vi "BRig_RT__Case_Exp__State_RewardPre__v10.vi"(0 "input_dataCurrent":u16[](array[numeric]), 7 "input_dataExp":u16[](array[numeric]), 9 "input_dataBlock":u16[][](array[numeric]), 11 "input_dataTrial":u16[][](array[numeric])) -> (1 "output_T_Reward":u16, 2 "output_c_nReward_total_R":u16, 3 "output_c_nReward_total_L":u16, 4 "output_dataCurrent":u16[](array[numeric]), 6 "output_DAB_L=L":bool, 8 "output_DAB_R=HighPorb":bool, 10 "output_dataBlock":u16[][](array[numeric]), 13 "output_c_nReward_total":u16, 14 "output_nReward":u16, 15 "output_dataTrial":u16[][](array[numeric]))   [LabVIEW 2014]
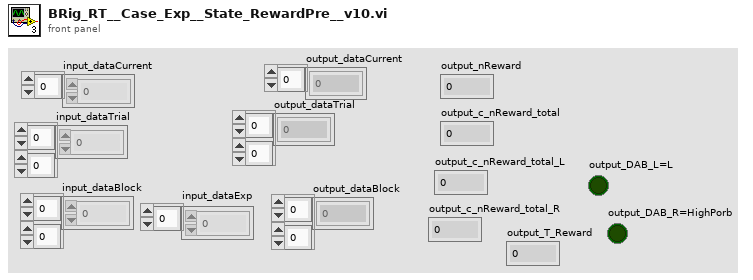
[diagram p1: front panel]
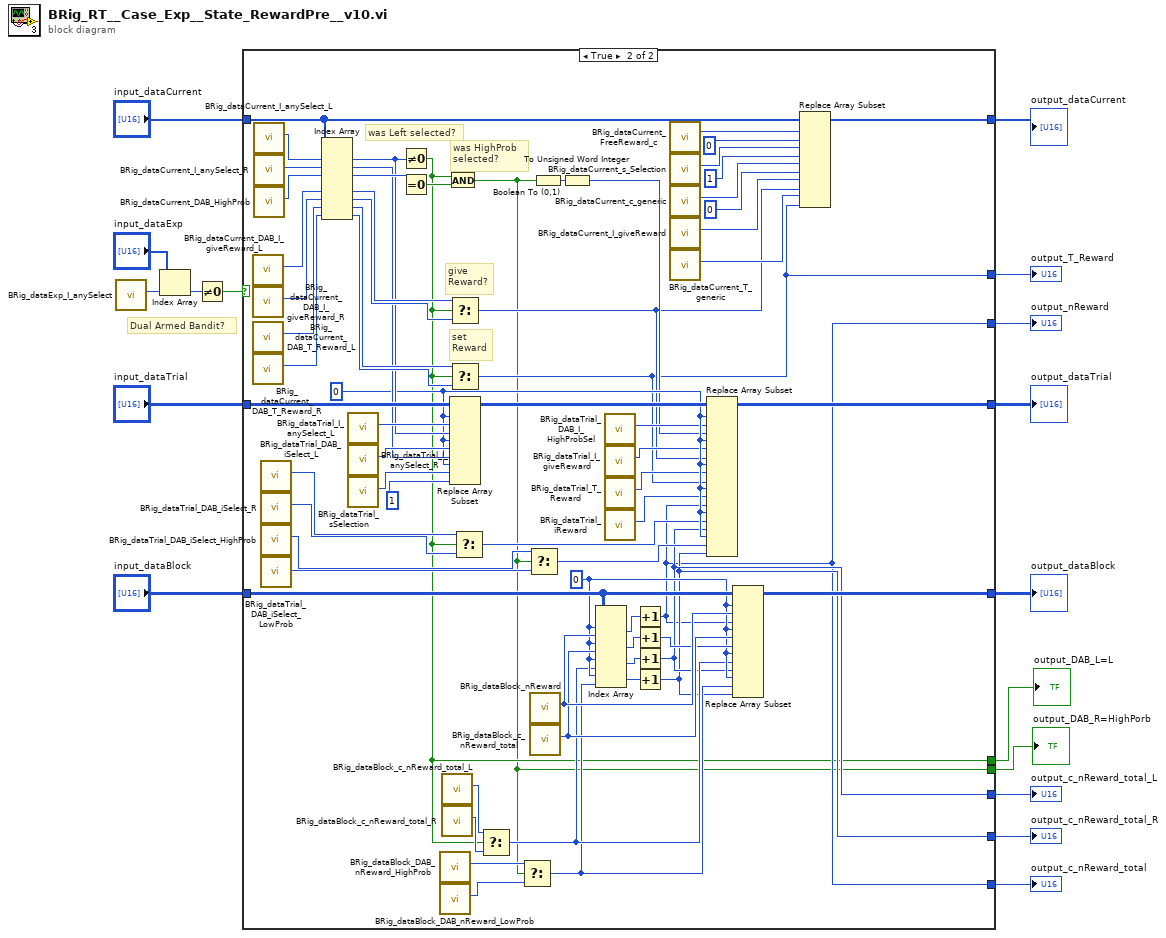
[diagram p0: block diagram]
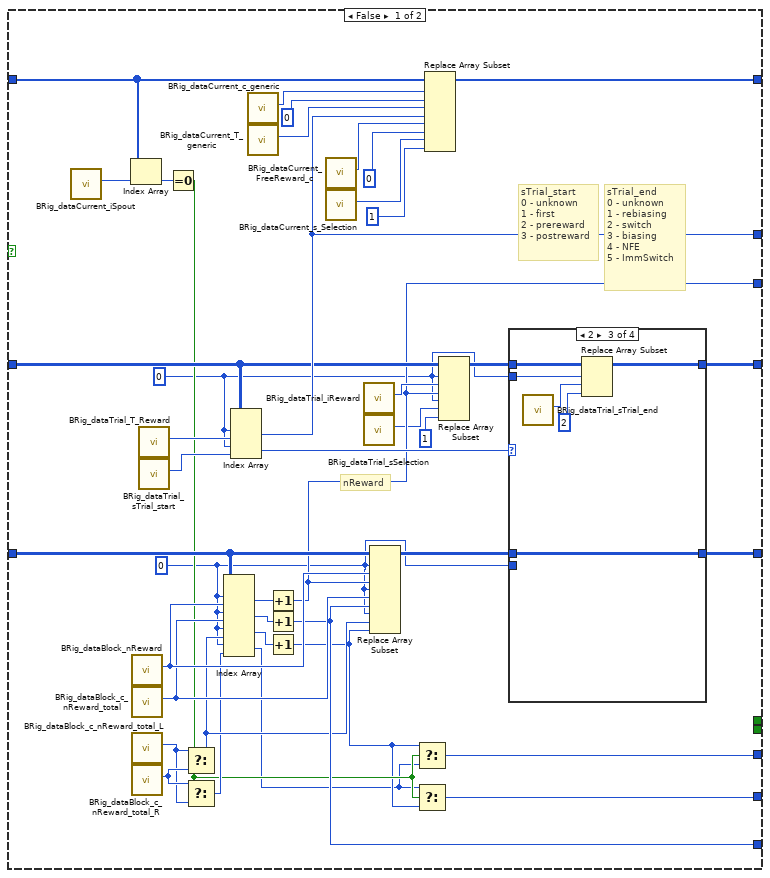
[diagram p2: hidden frame]
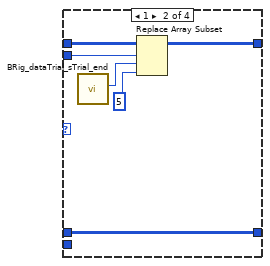
[diagram p4: hidden frame]
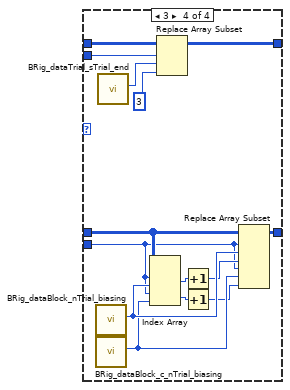
[diagram p5: hidden frame]
diagram:
  # "Dual Armed Bandit?"
  n1 = call "BRig_dataExp_I_anySelect.vi"() -> ("output_I_anySelect"=w10:i32)  [unwired: 11 in]
  n2 = Index Array(array="input_dataExp", index=w10) -> (element=w9:u16)
  n3 = Not Equal To 0?(x=w9) -> (x != 0?=w7:bool)
  n4 = case shown="True" w7 {
    tunnel: [w59 w155] -> w17
    tunnel: "input_dataCurrent" -> [w55 w146]
    tunnel: [w53 w93] -> w16
    tunnel: "input_dataBlock" -> [w52 w119]
    tunnel: [w47 w90] -> w15
    tunnel: "input_dataTrial" -> [w40 w128]
    tunnel: [w37 w90] -> w14
    tunnel: [w35 w116] -> w13
    tunnel: [w34 w117] -> w12
    tunnel: [w25 w92] -> w11
    tunnel: [w18 w91] -> w6
    tunnel: [_ w89] -> w2
    tunnel: [_ w88] -> w1
    frame False {
      w20 = 0
      w19 = 0
      # "nReward"
      # "sTrial_end\n0 - unknown\n1 - rebiasing\n2 - switch\n3 - biasing\n4 - NFE\n5 - ImmSwitch"
      # "sTrial_start\n0 - unknown\n1 - first\n2 - prereward\n3 - postreward"
      n5 = call "BRig_dataCurrent_iSpout.vi"() -> ("output_iSpout"=w46:i32)  [unwired: 11 in]
      n6 = Index Array(array=w55, index=w46) -> (element=w45:u16)
      n7 = call "BRig_dataBlock_nReward.vi"() -> ("output_nReward"=w51:i32)  [unwired: 11 in]
      n8 = call "BRig_dataBlock_c_nReward_total.vi"() -> ("output_nReward_total"=w48:i32)  [unwired: 11 in]
      n9 = call "BRig_dataBlock_c_nReward_total_L.vi"() -> ("output_nReward_total_L"=w30:i32)  [unwired: 11 in]
      n10 = call "BRig_dataBlock_c_nReward_total_R.vi"() -> ("output_nReward_total_R"=w31:i32)  [unwired: 11 in]
      n11 = call "BRig_dataTrial_T_Reward.vi"() -> ("output_T_Reward"=w54:i32)  [unwired: 11 in]
      n12 = call "BRig_dataTrial_sTrial_start.vi"() -> ("output_sTrial_start"=w42:i32)  [unwired: 11 in]
      n13 = Equal To 0?(x=w45) -> (x = 0?=w28:bool)
      n14 = Select(t=w30, s=w28, f=w31) -> (s? t:f=w43:i32)
      n15 = Select(t=w31, s=w28, f=w30) -> (s? t:f=w29:i32)
      n16 = Index Array(array=w52, index (row) #1=w19, index (col) #1=w51, index (row) #2=w19, index (col) #2=w48, index (row) #3=w19, index (col) #3=w43, index (row) #4=w19, index (col) #4=w29) -> (element #1=w50:u16, element #2=w49:u16, element #3=w44:u16, element #4=w26:u16)
      n17 = Index Array(array=w40, index (row) #1=w20, index (col) #1=w54, index (row) #2=w20, index (col) #2=w42) -> (element #1=w53:u16, element #2=w41:u16)
      n18 = call "BRig_dataCurrent_c_generic.vi"() -> ("output_count_generic"=w58:i32)  [unwired: 11 in]
      n19 = call "BRig_dataCurrent_T_generic.vi"() -> ("output_T_generic"=w57:i32)  [unwired: 11 in]
      n20 = Increment(x=w50) -> (x+1=w37:u16)
      n21 = Increment(x=w49) -> (x+1=w47:u16)
      n22 = Increment(x=w44) -> (x+1=w27:u16)
      n23 = call "BRig_dataCurrent_FreeReward_c.vi"() -> ("output_FreeReward_c"=w24:i32)  [unwired: 11 in]
      n24 = call "BRig_dataCurrent_s_Selection.vi"() -> ("output_s_Selection"=w22:i32)  [unwired: 11 in]
      n25 = call "BRig_dataTrial_iReward.vi"() -> ("output_iReward"=w38:i32)  [unwired: 11 in]
      n26 = call "BRig_dataTrial_sSelection.vi"() -> ("output_sSelection"=w33:i32)  [unwired: 11 in]
      n27 = Replace Array Subset(array=w52, new element #1=w37, index (row) #1=w19, index (col) #1=w51, new element #2=w47, index (row) #2=w19, index (col) #2=w48, new element #3=w27, index (row) #3=w19, index (col) #3=w43) -> (w36:u16[][])
      n28 = Select(t=w27, s=w28, f=w26) -> (s? t:f=w25:u16)
      n29 = Select(t=w26, s=w28, f=w27) -> (s? t:f=w18:u16)
      n30 = Replace Array Subset(array=w55, new element #1=u16 0 ("new element/subarray"), index #1=w58, new element #2=w53, index #2=w57, new element #3=u16 0 ("new element/subarray"), index #3=w24, new element #4=u16 1 ("new element/subarray"), index #4=w22) -> (w59:u16[])
      n31 = Replace Array Subset(array=w40, new element #1=w37, index (row) #1=w20, index (col) #1=w38, new element #2=u16 1 ("new element/subarray"), index (row) #2=w20, index (col) #2=w33) -> (w39:u16[][])
      n32 = case shown="2" w41 {
        tunnel: w39 -> [w61 w67 w73 w87]
        tunnel: w20 -> [_ w65 w71 w85]
        tunnel: [w61 w66 w72 w86] -> w34
        tunnel: w36 -> [w60 w62 w68 w81]
        tunnel: [w60 w62 w68 w82] -> w35
        tunnel: w19 -> [_ _ _ w77]
        frame 0, Default {
        }
        frame 1 {
          n33 = call "BRig_dataTrial_sTrial_end.vi"() -> ("output_sTrial_end"=w64:i32)  [unwired: 11 in]
          n34 = Replace Array Subset(array=w67, new element=u16 5 ("new element/subarray"), index (row)=w65, index (col)=w64) -> (w66:u16[][])
        }
        frame 2 {
          n35 = call "BRig_dataTrial_sTrial_end.vi"() -> ("output_sTrial_end"=w70:i32)  [unwired: 11 in]
          n36 = Replace Array Subset(array=w73, new element=u16 2 ("new element/subarray"), index (row)=w71, index (col)=w70) -> (w72:u16[][])
        }
        frame 3 {
          n37 = call "BRig_dataBlock_nTrial_biasing.vi"() -> ("output_nTrial_biasing"=w80:i32)  [unwired: 11 in]
          n38 = call "BRig_dataBlock_c_nTrial_biasing.vi"() -> ("output_c_nTrial_biasing"=w75:i32)  [unwired: 11 in]
          n39 = call "BRig_dataTrial_sTrial_end.vi"() -> ("output_sTrial_end"=w84:i32)  [unwired: 11 in]
          n40 = Index Array(array=w81, index (row) #1=w77, index (col) #1=w80, index (row) #2=w77, index (col) #2=w75) -> (element #1=w79:u16, element #2=w76:u16)
          n41 = Replace Array Subset(array=w87, new element=u16 3 ("new element/subarray"), index (row)=w85, index (col)=w84) -> (w86:u16[][])
          n42 = Increment(x=w79) -> (x+1=w78:u16)
          n43 = Increment(x=w76) -> (x+1=w74:u16)
          n44 = Replace Array Subset(array=w81, new element #1=w78, index (row) #1=w77, index (col) #1=w80, new element #2=w74, index (row) #2=w77, index (col) #2=w75) -> (w82:u16[][])
        }
      }
    }
    frame True {
      w115 = 0
      w102 = 0
      # "set\nReward"
      # "give\nReward?"
      # "was HighProb\nselected?"
      # "was Left selected?"
      n45 = call "BRig_dataCurrent_DAB_I_giveReward_L.vi"() -> ("output_DAB_I_giveReward_L"=w140:i32)  [unwired: 11 in]
      n46 = call "BRig_dataCurrent_DAB_I_giveReward_R.vi"() -> ("output_DAB_I_giveReward_R"=w139:i32)  [unwired: 11 in]
      n47 = call "BRig_dataCurrent_DAB_T_Reward_L.vi"() -> ("output_DAB_T_Reward_L"=w134:i32)  [unwired: 11 in]
      n48 = call "BRig_dataCurrent_DAB_T_Reward_R.vi"() -> ("output_DAB_T_Reward_R"=w133:i32)  [unwired: 11 in]
      n49 = call "BRig_dataCurrent_I_anySelect_L.vi"() -> ("output_IanySelect_L"=w145:i32)  [unwired: 11 in]
      n50 = call "BRig_dataCurrent_I_anySelect_R.vi"() -> ("output_IanySelect_R"=w144:i32)  [unwired: 11 in]
      n51 = call "BRig_dataCurrent_DAB_HighProb.vi"() -> ("output_DAB_HighProb"=w143:i32)  [unwired: 11 in]
      n52 = call "BRig_dataTrial_DAB_iSelect_L.vi"() -> ("output_DAB_iSelect_L"=w106:i32)  [unwired: 11 in]
      n53 = call "BRig_dataTrial_DAB_iSelect_R.vi"() -> ("output_DAB_iSelect_R"=w105:i32)  [unwired: 11 in]
      n54 = call "BRig_dataTrial_DAB_iSelect_HighProb.vi"() -> ("output_DAB_iSelect_HighProb"=w103:i32)  [unwired: 11 in]
      n55 = call "BRig_dataTrial_DAB_iSelect_LowProb.vi"() -> ("output_DAB_iSelect_LowProb"=w104:i32)  [unwired: 11 in]
      n56 = Index Array(array=w146, index #1=w145, index #2=w144, index #3=w143, index #5=w140, index #6=w139, index #7=w134, index #8=w133) -> (element #1=w127:u16, element #2=w126:u16, element #3=w142:u16, element #5=w138:u16, element #6=w137:u16, element #7=w136:u16, element #8=w135:u16)  [unwired: 1 in, 1 out]
      n57 = call "BRig_dataTrial_I_anySelect_L.vi"() -> ("output_I_allReward_L"=w132:i32)  [unwired: 11 in]
      n58 = call "BRig_dataTrial_I_anySelect_R.vi"() -> ("output_I_anySelect_R"=w131:i32)  [unwired: 11 in]
      n59 = call "BRig_dataTrial_sSelection.vi"() -> ("output_sSelection"=w130:i32)  [unwired: 11 in]
      n60 = Not Equal To 0?(x=w127) -> (x != 0?=w89:bool)
      n61 = Equal To 0?(x=w142) -> (x = 0?=w141:bool)
      n62 = call "BRig_dataBlock_DAB_nReward_HighProb.vi"() -> ("output_DAB_nReward_HighProb"=w112:i32)  [unwired: 11 in]
      n63 = call "BRig_dataBlock_DAB_nReward_LowProb.vi"() -> ("output_DAB_nReward_LowProb"=w111:i32)  [unwired: 11 in]
      n64 = call "BRig_dataBlock_c_nReward_total_L.vi"() -> ("output_nReward_total_L"=w114:i32)  [unwired: 11 in]
      n65 = call "BRig_dataBlock_c_nReward_total_R.vi"() -> ("output_nReward_total_R"=w113:i32)  [unwired: 11 in]
      n66 = And(x=w89, y=w141) -> (x .and. y?=w88:bool)
      n67 = Select(t=w138, s=w89, f=w137) -> (s? t:f=w94:u16)
      n68 = Select(t=w136, s=w89, f=w135) -> (s? t:f=w93:u16)
      n69 = Replace Array Subset(array=w128, new element #1=w127, index (row) #1=w102, index (col) #1=w132, new element #2=w126, index (row) #2=w102, index (col) #2=w131, new element #3=u16 1 ("new element/subarray"), index (row) #3=w102, index (col) #3=w130) -> (w125:u16[][])
      n70 = Select(t=w106, s=w89, f=w105) -> (s? t:f=w100:i32)
      n71 = Select(t=w114, s=w89, f=w113) -> (s? t:f=w108:i32)
      n72 = Select(t=w112, s=w88, f=w111) -> (s? t:f=w107:i32)
      n73 = Select(t=w103, s=w88, f=w104) -> (s? t:f=w101:i32)
      n74 = call "BRig_dataBlock_nReward.vi"() -> ("output_nReward"=w124:i32)  [unwired: 11 in]
      n75 = call "BRig_dataBlock_c_nReward_total.vi"() -> ("output_nReward_total"=w121:i32)  [unwired: 11 in]
      n76 = Boolean To (0,1)(Boolean=w88) -> (0, 1=w118:i16)
      n77 = To Unsigned Word Integer(number=w118) -> (unsigned 16bit integer=w95:u16)
      n78 = Index Array(array=w119, index (row) #1=w115, index (col) #1=w124, index (row) #2=w115, index (col) #2=w121, index (row) #3=w115, index (col) #3=w108, index (row) #4=w115, index (col) #4=w107) -> (element #1=w123:u16, element #2=w122:u16, element #3=w110:u16, element #4=w109:u16)
      n79 = call "BRig_dataTrial_DAB_I_HighProbSel.vi"() -> ("output_DAB_I_HighProbSel"=w96:i32)  [unwired: 11 in]
      n80 = call "BRig_dataTrial_I_giveReward.vi"() -> ("output_I_giveReward"=w97:i32)  [unwired: 11 in]
      n81 = call "BRig_dataTrial_T_Reward.vi"() -> ("output_T_Reward"=w98:i32)  [unwired: 11 in]
      n82 = call "BRig_dataTrial_iReward.vi"() -> ("output_iReward"=w99:i32)  [unwired: 11 in]
      n83 = Increment(x=w123) -> (x+1=w90:u16)
      n84 = Increment(x=w122) -> (x+1=w120:u16)
      n85 = Increment(x=w110) -> (x+1=w92:u16)
      n86 = Increment(x=w109) -> (x+1=w91:u16)
      n87 = call "BRig_dataCurrent_FreeReward_c.vi"() -> ("output_FreeReward_c"=w154:i32)  [unwired: 11 in]
      n88 = call "BRig_dataCurrent_s_Selection.vi"() -> ("output_s_Selection"=w152:i32)  [unwired: 11 in]
      n89 = call "BRig_dataCurrent_c_generic.vi"() -> ("output_count_generic"=w150:i32)  [unwired: 11 in]
      n90 = call "BRig_dataCurrent_I_giveReward.vi"() -> ("output_I_giveReward"=w148:i32)  [unwired: 11 in]
      n91 = call "BRig_dataCurrent_T_generic.vi"() -> ("output_T_generic"=w147:i32)  [unwired: 11 in]
      n92 = Replace Array Subset(array=w125, new element #1=w95, index (row) #1=w102, index (col) #1=w96, new element #2=w94, index (row) #2=w102, index (col) #2=w97, new element #3=w93, index (row) #3=w102, index (col) #3=w98, new element #4=w90, index (row) #4=w102, index (col) #4=w99, new element #5=w92, index (row) #5=w102, index (col) #5=w100, new element #6=w91, index (row) #6=w102, index (col) #6=w101) -> (w117:u16[][])
      n93 = Replace Array Subset(array=w119, new element #1=w90, index (row) #1=w115, index (col) #1=w124, new element #2=w120, index (row) #2=w115, index (col) #2=w121, new element #3=w92, index (row) #3=w115, index (col) #3=w108, new element #4=w91, index (row) #4=w115, index (col) #4=w107) -> (w116:u16[][])
      n94 = Replace Array Subset(array=w146, new element #1=u16 0 ("new element/subarray"), index #1=w154, new element #2=u16 1 ("new element/subarray"), index #2=w152, new element #3=u16 0 ("new element/subarray"), index #3=w150, new element #4=w94, index #4=w148, new element #5=w93, index #5=w147) -> (w155:u16[])
    }
  }
  "output_dataCurrent" <- w17
  "output_dataBlock" <- w13
  "output_dataTrial" <- w12
  "output_nReward" <- w14
  "output_c_nReward_total" <- w15
  "output_c_nReward_total_L" <- w11
  "output_c_nReward_total_R" <- w6
  "output_T_Reward" <- w16
  "output_DAB_L=L" <- w2
  "output_DAB_R=HighPorb" <- w1
